vi "oax_Extract From Curser.vi"(7 "Sound to Play":u16(ring) items=["Original", "Extracted", "Residue"], 8 "error in (no error)":errorcluster, 9 "Order waveform":waveform(dbl)[](array[waveform]), 10 "Vibration signals":waveform(dbl)[](array[waveform]), 11 "Order waveform":refnum<vi>) -> (0 "error out":errorcluster, 1 "Order Waveform Out":waveform(dbl)[](array[waveform]), 2 "waveform out":waveform(dbl), 3 "Duration":dbl, 5 "Fs":dbl)   [LabVIEW 2017]
uses:
  <vilib>/Waveform/WDTOps.llb/WDT Get Waveform Subset DBL.vi
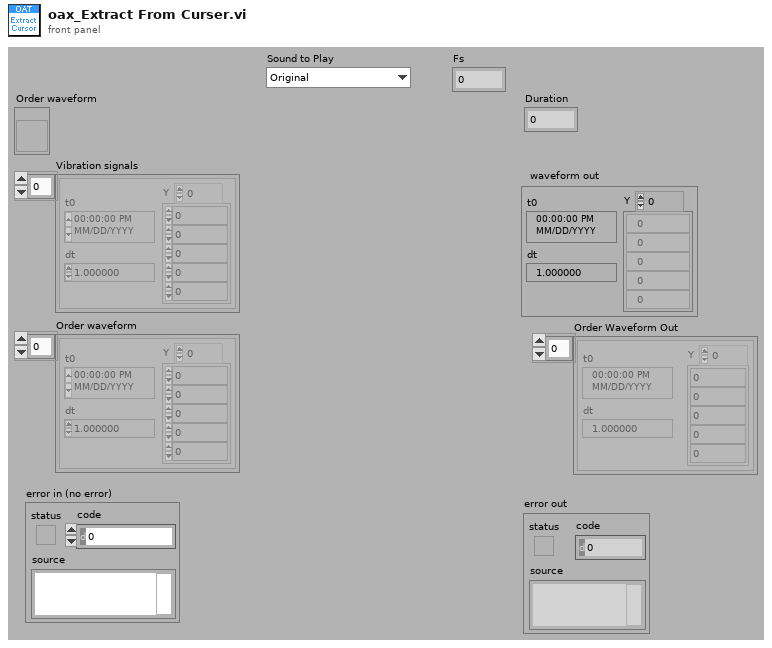
[diagram p1: front panel]
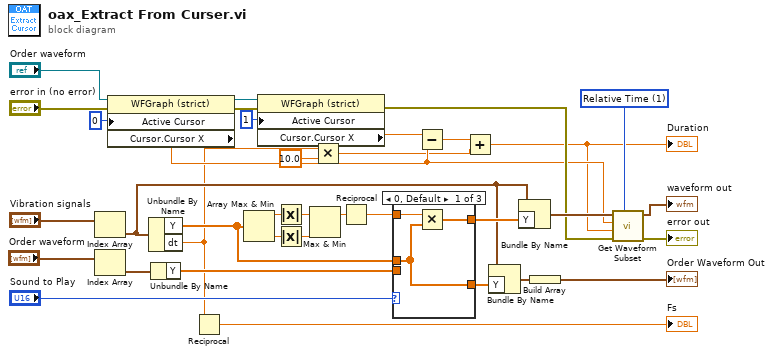
[diagram p0: block diagram]
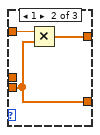
[diagram p2: hidden frame]
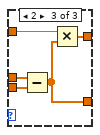
[diagram p3: hidden frame]
diagram:
  w7 = u16 1 items=["Samples", "Relative Time"] ("start/duration format")
  n1 = Index Array(array="Vibration signals") -> (element=w21:waveform(dbl))  [unwired: 1 in]
  n2 = Index Array(array="Order waveform") -> (element=w36:waveform(dbl))  [unwired: 1 in]
  n3 = property class="WFGraph (strict)"(reference="Order waveform", error in="error in (no error)", "Active Cursor"=u32 0) -> (reference out=w16:refnum<vi>, error out=w15:errorcluster, "Cursor.Cursor X"=w6:dbl)
  n4 = Unbundle By Name(w21) -> ("Y"=w27:dbl[], "dt"=w3:dbl)
  n5 = Unbundle By Name(w36) -> ("Y"=w26:dbl[])
  n6 = Reciprocal(x=w3) -> (1/x=→"Fs":dbl)
  n7 = Array Max & Min(array=w27) -> (max value=w31:dbl, min value=w30:dbl)  [unwired: 2 out]
  n8 = property class="WFGraph (strict)"(reference=w16, error in=w15, "Active Cursor"=u32 1) -> (error out=w12:errorcluster, "Cursor.Cursor X"=w13:dbl)  [unwired: 1 out]
  n9 = Absolute Value(x=w31) -> (abs(x)=w29:dbl)
  n10 = Absolute Value(x=w30) -> (abs(x)=w28:dbl)
  n11 = Max & Min(x=w29, y=w28) -> (max(x,y)=w32:dbl)  [unwired: 1 out]
  n12 = Multiply(x=w3, y=10.0) -> (x*y=w1:dbl)
  n13 = Reciprocal(x=w32) -> (1/x=w33:dbl)
  n14 = case shown="0, Default" "Sound to Play" {
    tunnel: w26 -> [_ w40 w46]
    tunnel: w27 -> [w37 _ w47]
    tunnel: w33 -> [w39 w42 w45]
    tunnel: [w38 w41 w44] -> w35
    tunnel: [w37 w40 w43] -> w25
    frame 0, Default {
      n15 = Multiply(x=w39, y=w37) -> (x*y=w38:dbl[])
    }
    frame 1 {
      n16 = Multiply(x=w42, y=w40) -> (x*y=w41:dbl[])
    }
    frame 2 {
      n17 = Subtract(x=w47, y=w46) -> (x-y=w43:dbl[])
      n18 = Multiply(x=w45, y=w43) -> (x*y=w44:dbl[])
    }
  }
  n19 = Subtract(x=w13, y=w6) -> (x-y=w4:dbl)
  n20 = Add(x=w4, y=w1) -> (x+y=w5:dbl)
  "Duration" <- w5
  n21 = Bundle By Name(cluster=w21, "Y"=w25) -> (w34:waveform(dbl))
  n22 = Bundle By Name(cluster=w21, "Y"=w35) -> (w23:waveform(dbl))
  n23 = Build Array(w34) -> (→"Order Waveform Out":waveform(dbl)[])
  n24 = call-poly <vilib>:"Get Waveform Subset.vi"("start/duration format"=w7, "error in (no error)"=w12, "duration"=w5, "start samples/time"=w6, "waveform in"=w23) -> ("error out"=→"error out":errorcluster, "waveform out"=→"waveform out":waveform(dbl))  [unwired: 1 in, 2 out]
